vi "Instrument Type ID.vi"() -> (1 "instrument type id":string="niScope")   [LabVIEW 2020, in "MeasurementLink niScope.lvlib" / "Instrument.lvclass"]
uses:
  Instrument.lvclass
  Instrument.lvclass/Instrument.ctl
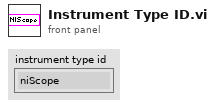
[diagram p1: front panel]
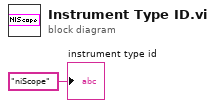
[diagram p0: block diagram]
diagram:
  "instrument type id" <- "niScope" ("instrument type id")
